vi "clearpath_read_serial.vi"(3 "Cluster In":T1, 4 "error in":errorcluster, 5 "VISA resource name in":refnum<visa-resource-name>) -> (0 "Cluster Out":T1, 1 "error out":errorcluster, 2 "VISA resource name out":refnum<visa-resource-name>)   [LabVIEW 2012, in "clearpath_interface.lvlib"]
doc: "Reads a serial port and splits up the data into valid CCP messages. Buffers must be provided as shown in the clearpath_crio demo interface to allow data to be stored properly."
uses:
  IGVC/Clearpath/Husky 2011/Teleop Robotics Project Folder/Husky/vi/clearpath_interface.lvlib
  cwrap_crio.dll
panel:
  out "RX String":string
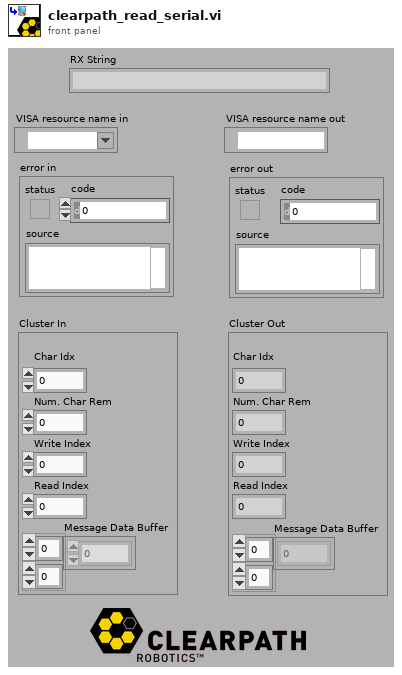
[diagram p1: front panel]
types:
  T1 = cluster{"\nChar Idx":u8, "Num. Char Rem":u8, "Write Index":u8, "Read Index":u8, "Message Data Buffer":u8[][]}
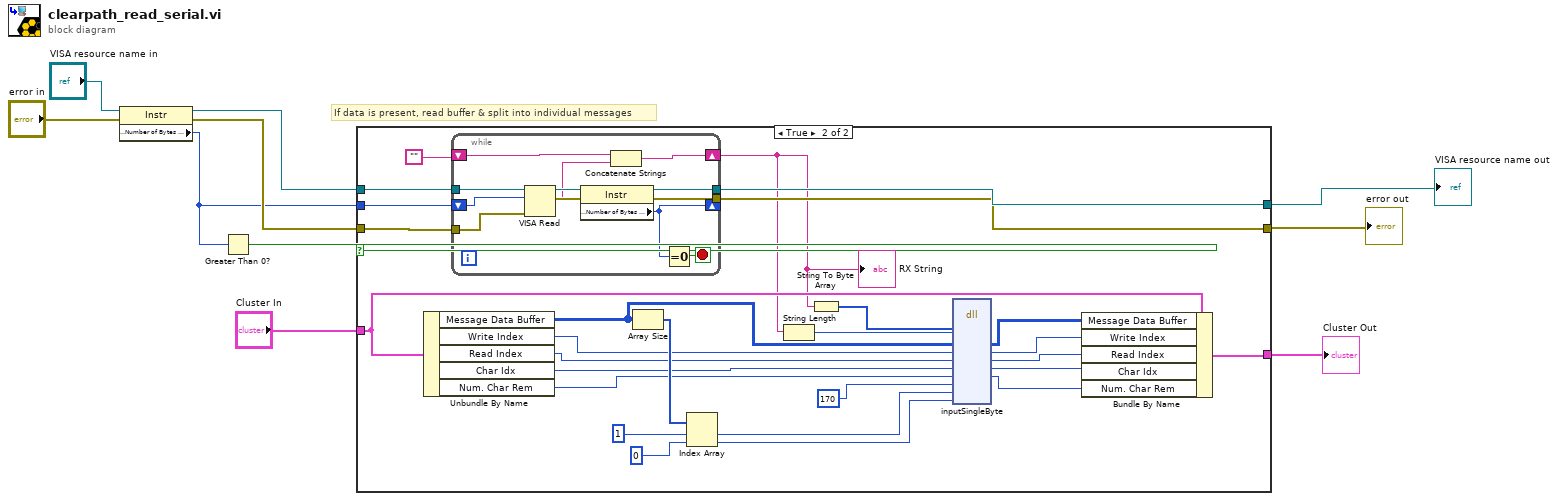
[diagram p0: block diagram]
diagram:
  # "If data is present, read buffer & split into individual messages"
  n1 = property class="Instr"(reference="VISA resource name in", error in="error in") -> (reference out=w5:refnum<visa-resource-name>, error out=w7:errorcluster, "Serial Settings:Number of Bytes at Serial Port"=w2:u32)
  n2 = Greater Than 0?(x=w2) -> (x > 0?=w8:bool)
  n3 = case shown="True" w8 {
    tunnel: [w13 w38] -> w1
    tunnel: w5 -> [w13 w40]
    tunnel: [w12 w37] -> w3
    tunnel: w7 -> [w12 w39]
    tunnel: w2 -> [_ w15]
    tunnel: "Cluster In" -> [w11 w36]
    tunnel: [w11 w35] -> w10
    frame False {
    }
    frame True {
      n4 = Unbundle By Name(w36) -> ("Message Data Buffer"=w23:u8[][], "Write Index"=w19:u8, "Read Index"=w20:u8, "Char Idx"=w21:u8, "Num. Char Rem"=w22:u8)
      n5 = while {
        tunnel: w40 -> [w52]
        tunnel: w39 -> [w51]
        tunnel: [w48] -> w38
        tunnel: [w47] -> w37
        shift-right: [w45] -> _
        shift-left: w15 -> [w44]
        shift-right: [w42] -> w16
        shift-left: "" -> [w43]
        stop <- w46 stop-if-true
        n6 = VISA Read(VISA resource name=w52, byte count=w44, error in (no error)=w51) -> (VISA resource name out=w50:refnum<visa-resource-name>, read buffer=w41:string, error out=w49:errorcluster)  [unwired: 1 out]
        n7 = property class="Instr"(reference=w50, error in=w49) -> (reference out=w48:refnum<visa-resource-name>, error out=w47:errorcluster, "Serial Settings:Number of Bytes at Serial Port"=w45:u32)
        n8 = Concatenate Strings(w43, w41) -> (w42:string)
        n9 = Equal To 0?(x=w45) -> (x = 0?=w46:bool)
      }
      "RX String" <- w16
      n10 = Array Size(array=w23) -> (size(s)=w31:i32[])
      n11 = Index Array(array=w31, index #1=1 ("index"), index #2=0 ("index")) -> (element #1=w17:i32, element #2=w18:i32)
      n12 = String Length(string=w16) -> (length=w29:i32)
      n13 = String To Byte Array(string=w16) -> (unsigned byte array=w34:u8[])
      n14 = dll-call lib="C:/Users/tebbeam/Documents/GitHub/IGVC-2013/Code/Project 1.0/Motors/Husky/cwrap_cRIO.*" fn="inputSingleByte"("new_bytes"=w34, "recv_len"=w29, "recv_buffer"=w23, "cur_write_buf"=w19, "cur_read_buf"=w20, "char_idx"=w21, "num_char_left"=w22, "SOH"=u8 170, "RECV_LEN"=w17, "NUM_BUF"=w18) -> ("recv_buffer"=w26:i8[][], "cur_write_buf"=w25:u8, "cur_read_buf"=w24:u8, "char_idx"=w27:u8, "num_char_left"=w28:u8)  [unwired: 9 in, 2 out]
      n15 = Bundle By Name(cluster=w36, "Message Data Buffer"=w26, "Write Index"=w25, "Read Index"=w24, "Char Idx"=w27, "Num. Char Rem"=w28) -> (w35:T1)
    }
  }
  "Cluster Out" <- w10
  "error out" <- w3
  "VISA resource name out" <- w1
